vi "Clear Hardware.vi"(2 "error in (no error)":errorcluster, 3 "Agilent ESG in":refnum<class "Agilent ESG.lvclass">) -> (0 "error out":errorcluster, 1 "Agilent ESG out":refnum<class "Agilent ESG.lvclass">)   [LabVIEW 2013, in "Agilent ESG.lvclass"]
doc: "This VI resets any necessary hardware so that the device will be ready for the next run."
uses:
  Agilent ESG.lvclass
  Device/Device.lvclass
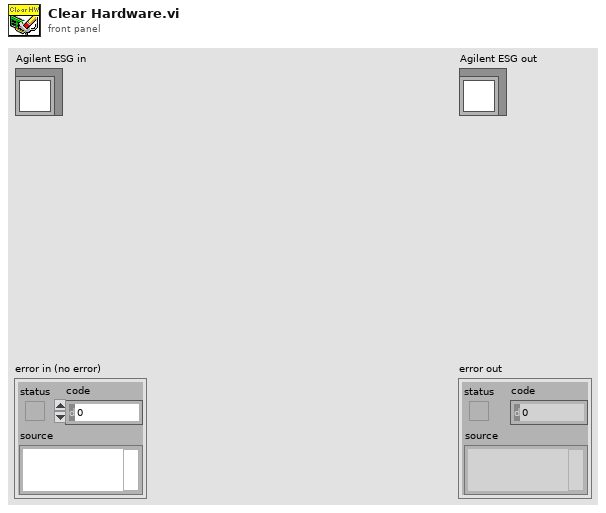
[diagram p1: front panel]
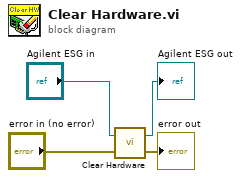
[diagram p0: block diagram]
diagram:
  n1 = call-parent "Clear Hardware.vi"("error in (no error)"="error in (no error)", "Device in"="Agilent ESG in") -> ("error out"=→"error out":errorcluster, "Device out"=→"Agilent ESG out":refnum<class "Agilent ESG.lvclass">)
